vi "getSenA.vi"(8 "error in (no error)":errorcluster, 11 "OptStateEsti in":refnum<class "OptStateEsti.lvclass">) -> (0 "error out":errorcluster, 2 "Matrix A":dbl[][](array[numeric]), 3 "OptStateEsti out":refnum<class "OptStateEsti.lvclass">)   [LabVIEW 2016, in "OptStateEsti.lvclass"]
uses:
  OptStateEsti.lvclass
  OptStateEsti.lvclass/OptStateEsti.ctl
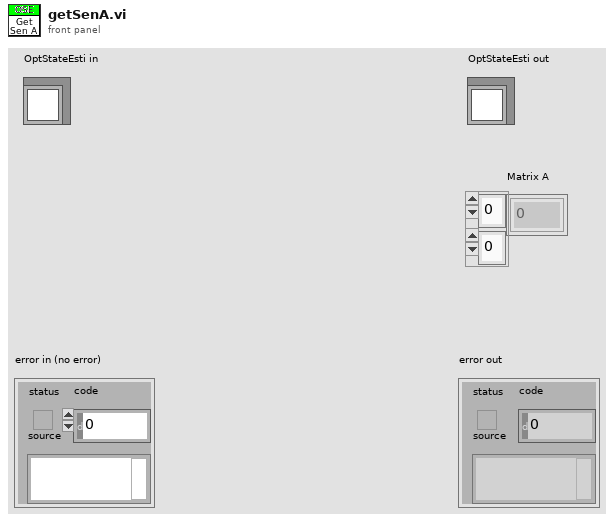
[diagram p1: front panel]
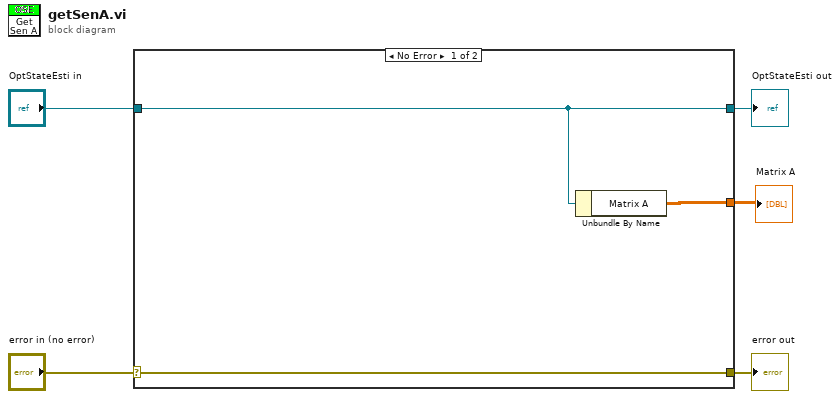
[diagram p0: block diagram]
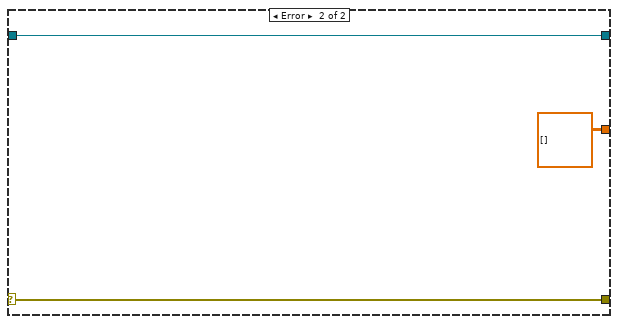
[diagram p2: hidden frame]
diagram:
  n1 = case shown="No Error" "error in (no error)" {
    selector: "error in (no error)" -> [w8 w11]
    tunnel: [w8 w11] -> w4
    tunnel: [w7 w10] -> w2
    tunnel: "OptStateEsti in" -> [w7 w10]
    tunnel: [w6 dbl[][] [] ("Matrix A")] -> w1
    frame No Error {
      n2 = Unbundle By Name(w7) -> ("Matrix A"=w6:dbl[][])
    }
    frame Error {
    }
  }
  "error out" <- w4
  "OptStateEsti out" <- w2
  "Matrix A" <- w1
